vi "WLAN_FrameAnalysis_BothMessages - Optimized.vi"(8 "error in (no error)":errorcluster, 11 "input cluster":cluster{"t0":dbl, "dt":dbl, "Y":cdb[]}) -> (0 "error out":errorcluster, 1 "Constellation":cdb[](graph), 2 "Modulation parameter":T1, 3 "SC Bits":i8[](array[numeric]), 4 "Frequency offset":dbl, 5 "SIG valid?":bool, 7 "Base Bits":i8[](array[numeric]))   [LabVIEW 2022 SP3]
panel:
  out "x+y":dbl
  out "Frequency offset(LTF)":dbl
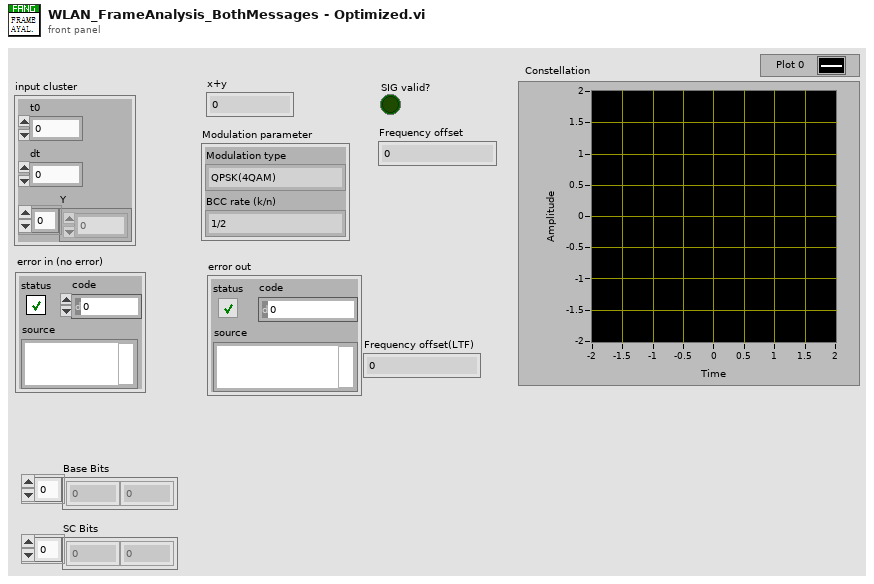
[diagram p1: front panel]
types:
  T1 = cluster{"Modulation type":enum16{"QPSK(4QAM)", "64QAM", "16QAM", "BPSK"}, "BCC rate (k/n)":enum16{"1/2", "2/3", "3/4"}}
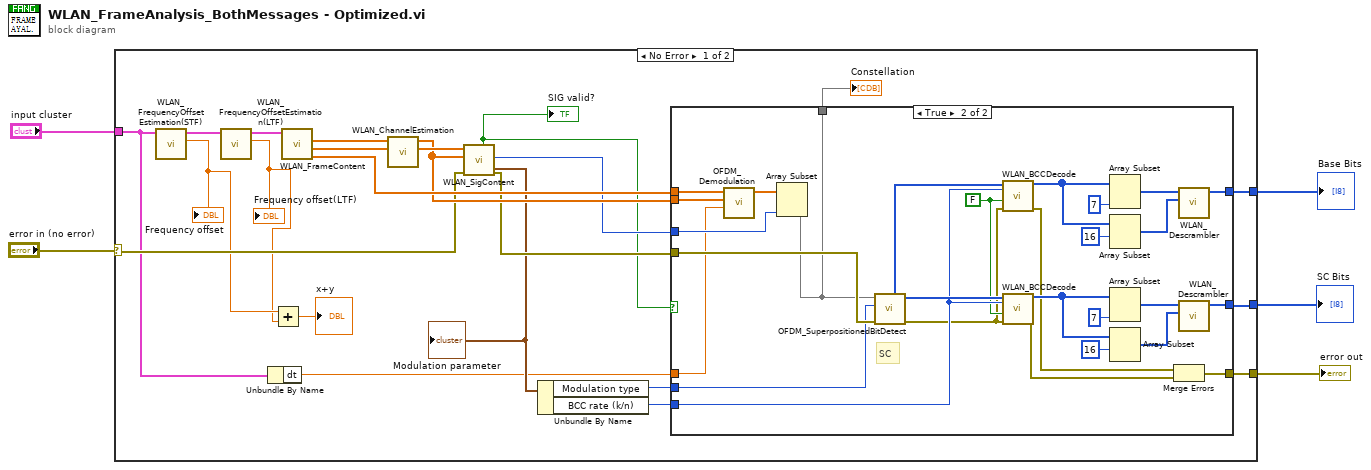
[diagram p0: block diagram]
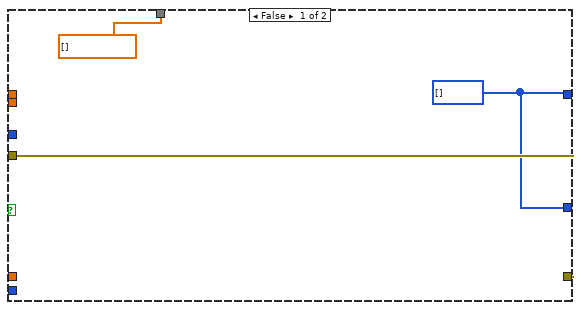
[diagram p2: hidden frame]
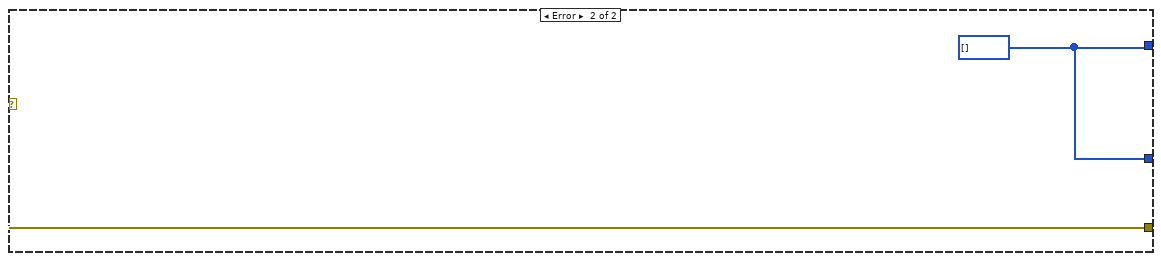
[diagram p3: hidden frame]
diagram:
  n1 = case shown="No Error" "error in (no error)" {
    selector: "error in (no error)" -> [w14 w60]
    tunnel: "input cluster" -> [w8 _]
    tunnel: [w21 w60] -> w4
    tunnel: [w20 w59] -> w3
    tunnel: [w6 w59] -> w1
    frame No Error {
      n2 = call "WLAN_FrequencyOffsetEstimation(STF).vi"("output cluster"=w8) -> ("Frequency offset(STF)"=w12:dbl, "output cluster 2"=w13:cluster{"t0":dbl, "dt":dbl, "Y":cdb[]})  [unwired: 8 in]
      "Frequency offset" <- w12
      n3 = call "WLAN_FrequencyOffsetEstimation(LTF).vi"("input cluster"=w13) -> ("Frequency offset(LTF)"=w11:dbl, "output cluster"=w9:cluster{"t0":dbl, "dt":dbl, "Y":cdb[]})  [unwired: 9 in]
      "Frequency offset(LTF)" <- w11
      n4 = Unbundle By Name(w8) -> ("dt"=w7:dbl)
      n5 = Add(x=w12, y=w11) -> (x+y=→"x+y":dbl)
      n6 = call "WLAN_FrameContent.vi"("Input cluster"=w9) -> ("DATA"=w27:cdb[], "SIG"=w25:cdb[], "LTF"=w26:cdb[])  [unwired: 7 in, 1 out]
      n7 = call "WLAN_ChannelEstimation.vi"("LTF"=w26) -> ("Frequency estimation"=w24:cdb[])  [unwired: 10 in]
      n8 = call "WLAN_SigContent.vi"("error in (no error)"=w14, "Frequency channel estimation"=w24, "SIG"=w25) -> ("error out"=w23:errorcluster, "Symbol numbers"=w22:i32, "Modulation parameter"=w19:T1, "SIG valid?"=w15:bool)  [unwired: 3 in, 2 out]
      "Modulation parameter" <- w19
      "SIG valid?" <- w15
      n9 = Unbundle By Name(w19) -> ("Modulation type"=w18:enum16{"QPSK(4QAM)", "64QAM", "16QAM", "BPSK"}, "BCC rate (k/n)"=w17:enum16{"1/2", "2/3", "3/4"})
      n10 = case shown="True" w15 {
        tunnel: w27 -> [_ w58]
        tunnel: [w30 w34] -> w21
        tunnel: w24 -> [_ w56]
        tunnel: w23 -> [w30 w55]
        tunnel: w22 -> [_ w54]
        tunnel: w18 -> [_ w53]
        tunnel: [w28 w45] -> w20
        tunnel: w17 -> [_ w37]
        tunnel: [cdb[] [] w48] -> w16
        tunnel: w7 -> [_ w44]
        tunnel: [w28 w35] -> w6
        frame False {
          w28 = i8[] [] ("scrambled bits")
        }
        frame True {
          w36 = FALSE ("need add zeros?")
          # "SC"
          n11 = call "OFDM_Demodulation.vi"("sampling period"=w44, "Frequency channel estimation"=w56, "Input sequence"=w58) -> ("Output sequence"=w57:cdb[])  [unwired: 7 in, 1 out]
          n12 = Array Subset(array=w57, length=w54) -> (w48:cdb[])  [unwired: 1 in]
          n13 = call "OFDM_SuperpositionedBitDetect.vi"("Input symbols"=w48, "Modulation type"=w53, "error in (no error)"=w55) -> ("Base Bits"=w38:i8[], "SC Bits"=w47:i8[], "error out"=w31:errorcluster)  [unwired: 4 in, 1 out]
          n14 = call "WLAN_BCCDecode.vi"("error in (no error)"=w31, "need add zeros?"=w36, "BCC rate (k/n)"=w37, "input bit stream"=w38) -> ("error out"=w32:errorcluster, "output bit stream"=w43:i8[])  [unwired: 6 in]
          n15 = call "WLAN_BCCDecode.vi"("error in (no error)"=w31, "need add zeros?"=w36, "BCC rate (k/n)"=w37, "input bit stream"=w47) -> ("error out"=w33:errorcluster, "output bit stream"=w46:i8[])  [unwired: 6 in]
          n16 = Array Subset(array=w43, length=7) -> (w42:i8[])  [unwired: 1 in]
          n17 = Array Subset(array=w43, index=16) -> (w41:i8[])  [unwired: 1 in]
          n18 = Array Subset(array=w46, length=7) -> (w49:i8[])  [unwired: 1 in]
          n19 = Array Subset(array=w46, index=16) -> (w50:i8[])  [unwired: 1 in]
          n20 = Merge Errors(w32, w33) -> (w34:errorcluster)
          n21 = call "WLAN_Descrambler.vi"("scrambler initial bits"=w42, "data bits"=w41) -> ("scrambled bits"=w35:i8[])  [unwired: 7 in]
          n22 = call "WLAN_Descrambler.vi"("scrambler initial bits"=w49, "data bits"=w50) -> ("scrambled bits"=w45:i8[])  [unwired: 7 in]
        }
      }
      "Constellation" <- w16
    }
    frame Error {
      w59 = i8[] [] ("scrambled bits")
    }
  }
  "error out" <- w4
  "SC Bits" <- w3
  "Base Bits" <- w1
